vi "SPI Clock.vi"(8 "Count?":bool, 10 "Max Value":u16, 11 "Clock Select":T1) -> (3 "Enable Out":bool)   [LabVIEW 2015]
uses:
  SPI Clock Select.ctl
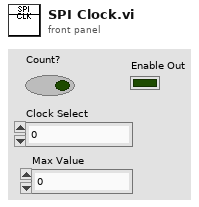
[diagram p1: front panel]
types:
  T1 = typedef "SPI Clock Select.ctl" = fxp<+,2,2>
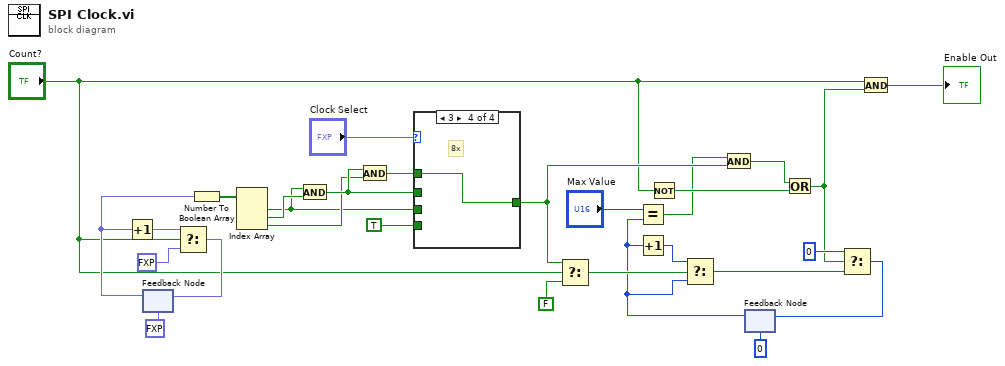
[diagram p0: block diagram]
diagram:
  n1 = feedback #1(fxp<+,3,3> 0.0 ("y")) -> (w18:fxp<+,3,3>)
  n2 = Increment(x=w18) -> (x+1=w26:fxp<+,3,3>)
  n3 = Select(t=w26, s="Count?", f=fxp<+,3,3> 0.0 ("y")) -> (s? t:f=w27:fxp<+,3,3>)
  n4 = feedback-in #1(w27) -> ()
  n5 = Number To Boolean Array(number=w18) -> (Boolean array=w19:bool[])
  n6 = Index Array(array=w19) -> (element #1=w20:bool, element #2=w21:bool, element #3=w22:bool)  [unwired: 3 in]
  n7 = And(x=w20, y=w21) -> (x .and. y?=w23:bool)
  n8 = And(x=w23, y=w22) -> (x .and. y?=w24:bool)
  n9 = case shown="3" "Clock Select" {
    tunnel: w20 -> [_ w31 _ _]
    tunnel: w23 -> [_ _ w32 _]
    tunnel: w24 -> [_ _ _ w33]
    tunnel: TRUE -> [w30 _ _ _]
    tunnel: [w30 w31 w32 w33] -> w7
    frame 0, Default {
      # "1x"
    }
    frame 1 {
      # "2x"
    }
    frame 2 {
      # "4x"
    }
    frame 3 {
      # "8x"
    }
  }
  n10 = Select(t=w7, s="Count?", f=FALSE) -> (s? t:f=w15:bool)
  n11 = Not(x="Count?") -> (.not. x?=w8:bool)
  n12 = feedback #2(u16 0 ("Max Value")) -> (w3:u16)
  n13 = Equal?(x="Max Value", y=w3) -> (x = y?=w4:bool)
  n14 = Increment(x=w3) -> (x+1=w14:u16)
  n15 = Select(t=w14, s=w15, f=w3) -> (s? t:f=w9:u16)
  n16 = And(x=w4, y=w7) -> (x .and. y?=w6:bool)
  n17 = Or(x=w6, y=w8) -> (x .or. y?=w5:bool)
  n18 = Select(t=u16 0 ("Max Value"), s=w5, f=w9) -> (s? t:f=w11:u16)
  n19 = feedback-in #2(w11) -> ()
  n20 = And(x="Count?", y=w5) -> (x .and. y?=→"Enable Out":bool)
